vi "set_pid_configuration.vi"(8 "error in (no error)":errorcluster, 9 "Disable adaptive control":bool, 10 "Control action":string(combo)="0", 11 "VISA Refnum in":refnum<visa-resource-name>) -> (0 "error out":errorcluster, 3 "VISA Refnum out":refnum<visa-resource-name>)   [LabVIEW 2018]
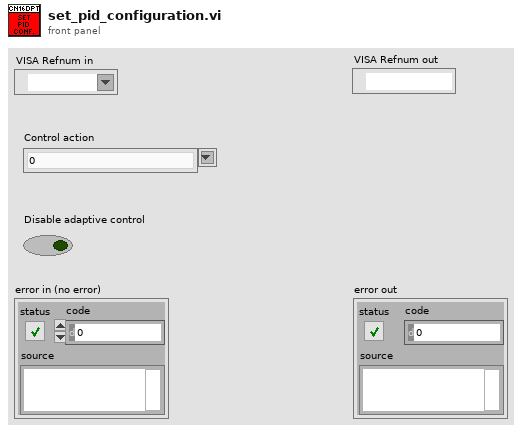
[diagram p1: front panel]
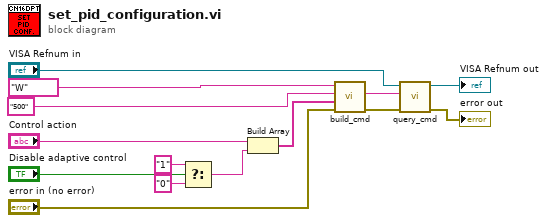
[diagram p0: block diagram]
diagram:
  n1 = Select(t="1", s="Disable adaptive control", f="0") -> (s? t:f=w2:string)
  n2 = Build Array("Control action", w2) -> (w1:string[])
  n3 = call "build_cmd.vi"("error in (no error)"="error in (no error)", "Parameter list"=w1, "Command ID"="500", "Command class"="W") -> ("error out"=w9:errorcluster, "Command"=w8:string)  [unwired: 6 in]
  n4 = call "query_cmd.vi"("error in (no error)"=w9, "Command"=w8, "VISA resource name"="VISA Refnum in") -> ("error out"=→"error out":errorcluster, "VISA resource name out"=→"VISA Refnum out":refnum<visa-resource-name>)  [unwired: 6 in, 1 out]
